vi "1.3.15 - New Lidar Transform.vi"(0 "Lidar Distance Value":u16, 1 "Lidar Scan Angle":u8, 2 "Lidar Forward Pos (X)":u8, 3 "Lidar Left/Right Pos (Y)":u8, 4 "Lidar Tilt Angle":i8, 5 "Lidar Height (Z)":u8) -> (6 "X obstacle":fxp<+/-,48,18> format="%.36g", 7 "Y obstacle":fxp<+/-,48,18> format="%.36g", 8 "Z obstacle":fxp<+/-,33,18> format="%.21g")   [LabVIEW 2010]
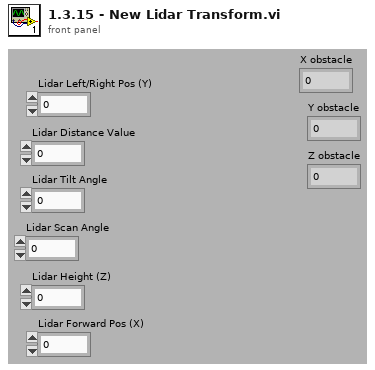
[diagram p1: front panel]
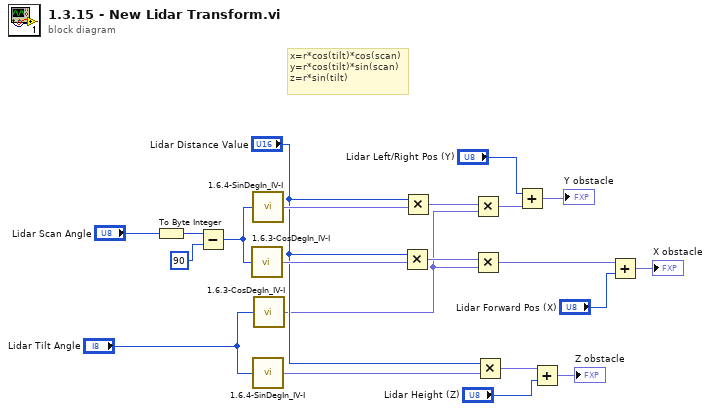
[diagram p0: block diagram]
diagram:
  # "x=r*cos(tilt)*cos(scan)\ny=r*cos(tilt)*sin(scan)\nz=r*sin(tilt)"
  n1 = To Byte Integer(number="Lidar Scan Angle") -> (8bit integer=w19:i8)
  n2 = Subtract(x=w19, y=i8 90) -> (x-y=w18:i8)
  n3 = call "1.6.3-CosDegIn_IV-I.vi"("theta"=w18) -> ("Numeric"=w16:fxp<+/-,16,1>)
  n4 = call "1.6.4-SinDegIn_IV-I.vi"("theta"=w18) -> ("Numeric"=w15:fxp<+/-,16,1>)
  n5 = call "1.6.4-SinDegIn_IV-I.vi"("theta"="Lidar Tilt Angle") -> ("Numeric"=w2:fxp<+/-,16,1>)
  n6 = call "1.6.3-CosDegIn_IV-I.vi"("theta"="Lidar Tilt Angle") -> ("Numeric"=w1:fxp<+/-,16,1>)
  n7 = Multiply(x="Lidar Distance Value", y=w16) -> (x*y=w13:fxp<+/-,32,17>)
  n8 = Multiply(x="Lidar Distance Value", y=w15) -> (x*y=w14:fxp<+/-,32,17>)
  n9 = Multiply(x=w14, y=w1) -> (x*y=w5:fxp<+/-,47,17>)
  n10 = Multiply(x=w13, y=w1) -> (x*y=w11:fxp<+/-,47,17>)
  n11 = Multiply(x="Lidar Distance Value", y=w2) -> (x*y=w8:fxp<+/-,32,17>)
  n12 = Add(x="Lidar Left/Right Pos (Y)", y=w5) -> (x+y=→"Y obstacle":fxp<+/-,48,18>)
  n13 = Add(x=w8, y="Lidar Height (Z)") -> (x+y=→"Z obstacle":fxp<+/-,33,18>)
  n14 = Add(x=w11, y="Lidar Forward Pos (X)") -> (x+y=→"X obstacle":fxp<+/-,48,18>)
